vi "Read Write Delay.vi"(7 "Skip delay? (F)":bool, 8 "error in":errorcluster) -> (0 "error out":errorcluster)   [LabVIEW 2020, in "QuPMXdriver.lvlib"]
doc: "Delay required between sending command and reading output.\nIn case of error the delay is always skipped."
uses:
  QuPMXdriver.lvlib
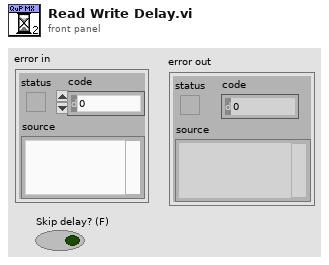
[diagram p1: front panel]
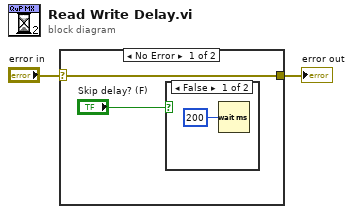
[diagram p0: block diagram]
diagram:
  n1 = case shown="No Error" "error in" {
    selector: "error in" -> [w3 w6]
    tunnel: [w3 w6] -> w1
    frame No Error {
      n2 = case shown="False" "Skip delay? (F)" {
        frame False {
          n3 = Wait (ms)(milliseconds to wait=u32 200) -> ()  [unwired: 1 out]
        }
        frame True {
        }
      }
    }
    frame Error {
    }
  }
  "error out" <- w1
